vi "Gen Machine Code.vi"(8 "error in (no error)":errorcluster, 11 "[MV] Key Certify in":refnum<class "[MV] Key Certify.lvclass">) -> (0 "error out":errorcluster, 3 "[MV] Key Certify out":refnum<class "[MV] Key Certify.lvclass">)   [LabVIEW 2020, in "[MV] Key Certify.lvlib" / "[MV] Key Certify.lvclass"]
uses:
  [MV] Key Certify.lvclass
  [MV] Key Certify.lvclass/[MV] Key Certify.ctl
  <vilib>/YU/Encrypt/MD5/MD5.lvclass
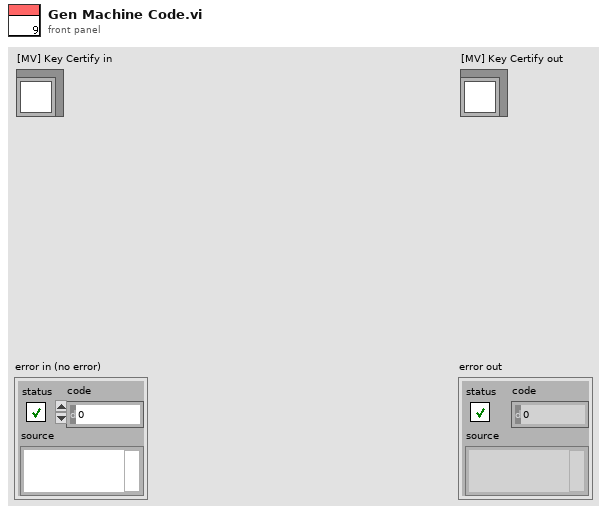
[diagram p1: front panel]
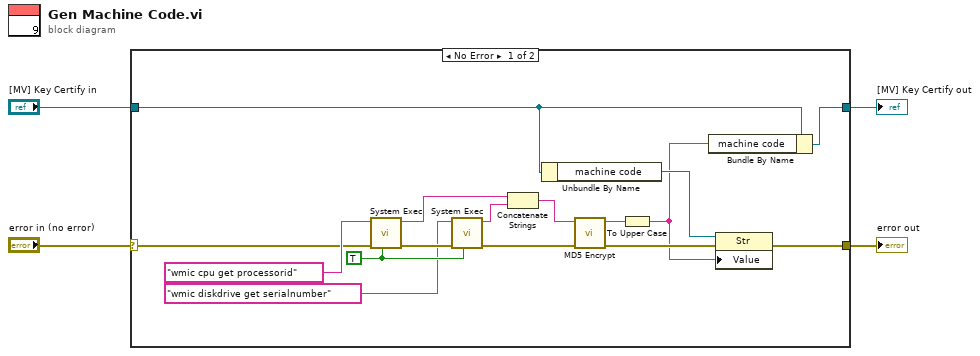
[diagram p0: block diagram]
diagram:
  n1 = case shown="No Error" "error in (no error)" {
    selector: "error in (no error)" -> [w14 w22]
    tunnel: [w5 w22] -> w3
    tunnel: [w10 w21] -> w1
    tunnel: "[MV] Key Certify in" -> [w9 w21]
    frame No Error {
      w18 = TRUE ("run minimized? (F)")
      n2 = call <vilib>:"System Exec.vi"("run minimized? (F)"=w18, "error in (no error)"=w14, "command line"="wmic cpu get processorid") -> ("error out"=w19:errorcluster, "standard output"=w15:string)  [unwired: 5 in, 2 out]
      n3 = call <vilib>:"System Exec.vi"("run minimized? (F)"=w18, "error in (no error)"=w19, "command line"="wmic diskdrive get serialnumber") -> ("error out"=w13:errorcluster, "standard output"=w17:string)  [unwired: 5 in, 2 out]
      n4 = Concatenate Strings(w15, w17) -> (w12:string)
      n5 = Unbundle By Name(w9) -> ("machine code"=w7:refnum<vi>)
      n6 = call <vilib>:"MD5 Encrypt.vi"("error in (no error)"=w13, "data"=w12) -> ("error out"=w8:errorcluster, "encrypted data"=w11:string)  [unwired: 8 in]
      n7 = To Upper Case(1:w11) -> (0:w6:string)
      n8 = Bundle By Name(cluster=w9, "machine code"=w6) -> (w10:refnum<class "[MV] Key Certify.lvclass">)
      n9 = property class="Str"(reference=w7, error in=w8, "Value"=w6) -> (error out=w5:errorcluster)  [unwired: 1 out]
    }
    frame Error {
    }
  }
  "error out" <- w3
  "[MV] Key Certify out" <- w1
